vi "TestPowerMeasure.vi"(3 "error in (no error)":errorcluster, 5 "OphirComRef":refnum<k7>) -> (0 "error out":errorcluster, 2 "SerialNumber":string)   [LabVIEW 2012]
uses:
  <vilib>/Analysis/baseanly.llb/Mean (DBL).vi
  <vilib>/Analysis/NI_AALBase.lvlib
panel:
  in  "Measure":bool
  in  "Stop":bool
  out "arrayValue":variant
  out "Array 2":dbl[][](array[numeric])
  out "x != 0?":bool
  out "Array":dbl[](array[numeric])
  out "Errors":dbl[](array[numeric])
  out "mean":dbl format="%.6g"
  out "median":dbl format="%.6g"
  in  "Wavelength":dbl
  in  "Samples":i32
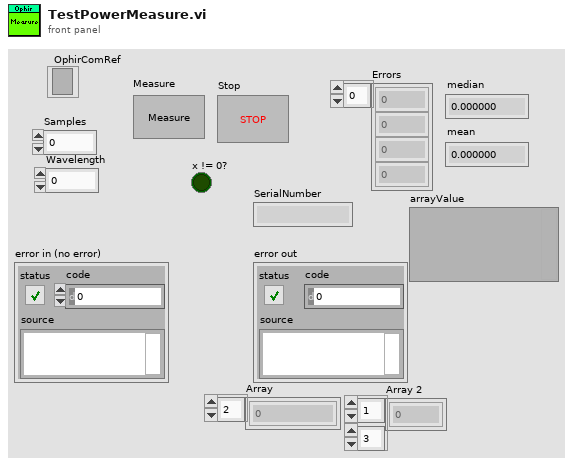
[diagram p1: front panel]
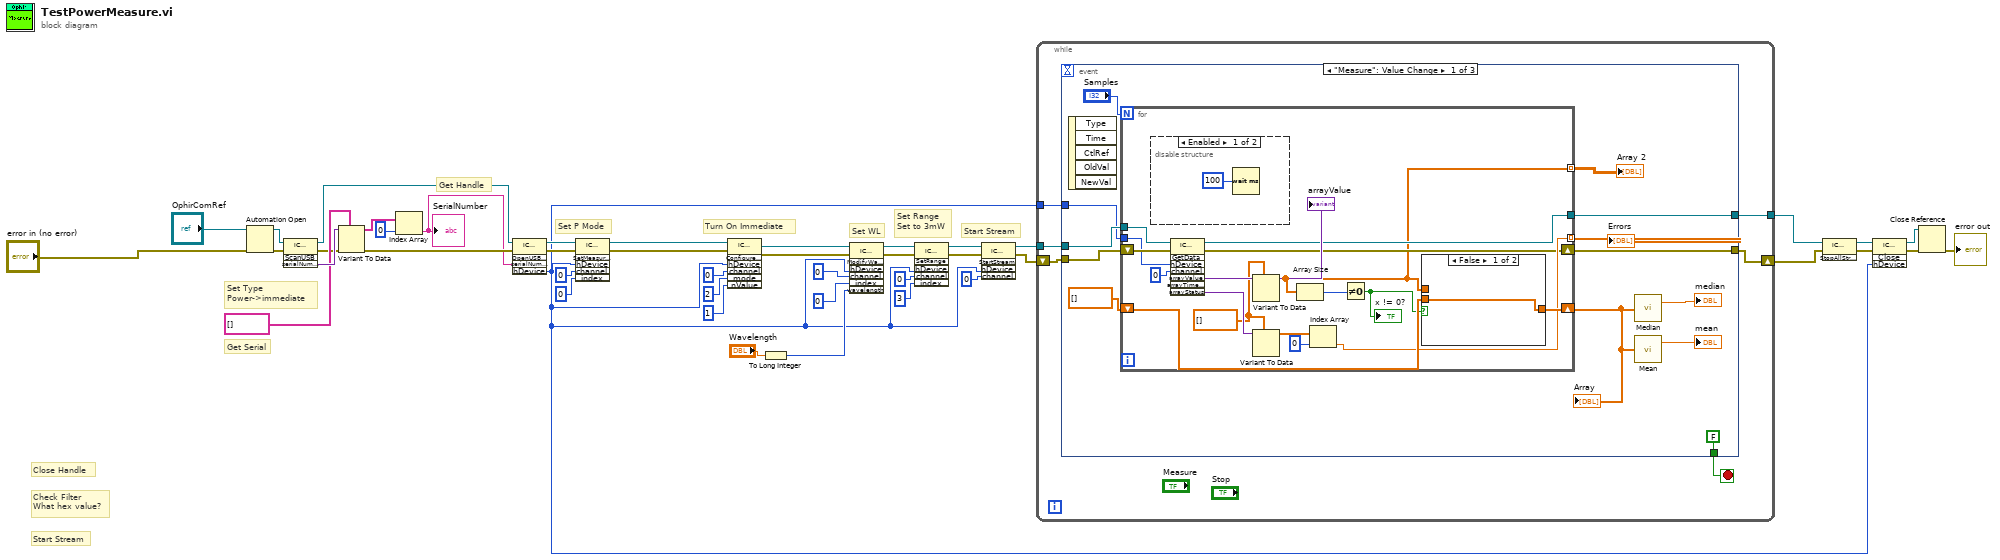
[diagram p0: block diagram]
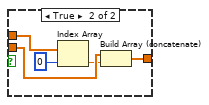
[diagram p3: hidden frame]
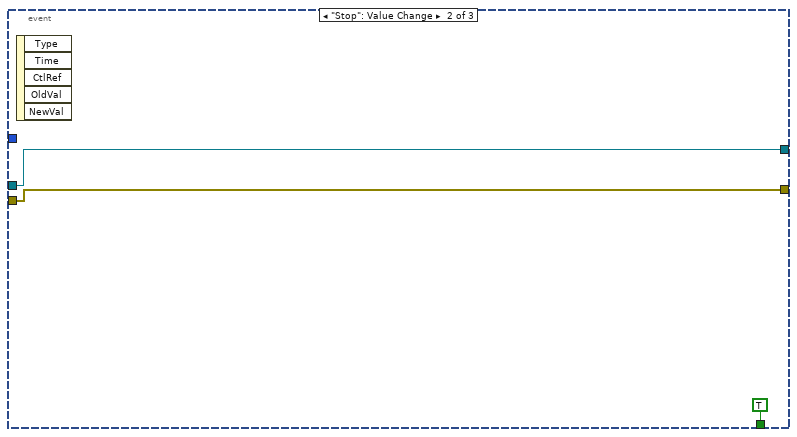
[diagram p4: hidden frame]
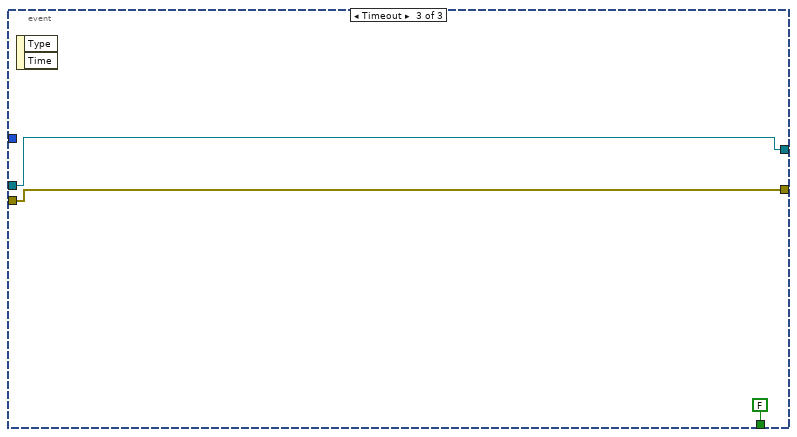
[diagram p5: hidden frame]
diagram:
  # "Start Stream"
  # "Set P Mode"
  # "Turn On Immediate"
  # "Set Type\nPower->immediate"
  # "Close Handle"
  # "Set Range\nSet to 3mW"
  # "Check Filter\nWhat hex value?"
  # "Start Stream"
  # "Get Handle"
  # "Get Serial"
  # "Set WL"
  n1 = Automation Open(error in (no error)="error in (no error)", Automation Refnum="OphirComRef") -> (Automation Refnum=w42:refnum<k7>, error out=w37:errorcluster)  [unwired: 2 in]
  n2 = invoke class="ICoLMMeasurement" method="ScanUSB"(reference=w42, error in=w37) -> (reference out=w34:refnum<k7>, error out=w38:errorcluster, "serialNumbers"=w41:variant)  [unwired: 2 in, 1 out]
  n3 = Variant To Data(error in=w38, type=string[] [], Variant=w41) -> (data=w39:string[], error out=w33:errorcluster)
  n4 = Index Array(array=w39, index=0) -> (element=w32:string)
  "SerialNumber" <- w32
  n5 = invoke class="ICoLMMeasurement" method="OpenUSBDevice"(reference=w34, error in=w33, "serialNumber"=w32) -> (reference out=w18:refnum<k7>, error out=w2:errorcluster, "hDevice"=w1:i32)  [unwired: 2 in, 2 out]
  n6 = invoke class="ICoLMMeasurement" method="SetMeasurementMode"(reference=w18, error in=w2, "hDevice"=w1, "channel"=0, "index"=0) -> (reference out=w4:refnum<k7>, error out=w3:errorcluster)  [unwired: 1 in, 4 out]
  n7 = invoke class="ICoLMMeasurement" method="ConfigureStreamMode"(reference=w4, error in=w3, "hDevice"=w1, "channel"=0 ("mode"), "mode"=2, "nValue"=1) -> (reference out=w7:refnum<k7>, error out=w6:errorcluster)  [unwired: 1 in, 5 out]
  n8 = To Long Integer(number="Wavelength") -> (32bit integer=w26:i32)
  n9 = invoke class="ICoLMMeasurement" method="ModifyWavelength"(reference=w7, error in=w6, "hDevice"=w1, "channel"=0, "index"=0, "wavelength"=w26) -> (reference out=w24:refnum<k7>, error out=w23:errorcluster)  [unwired: 1 in, 5 out]
  n10 = invoke class="ICoLMMeasurement" method="SetRange"(reference=w24, error in=w23, "hDevice"=w1, "channel"=0, "index"=3) -> (reference out=w13:refnum<k7>, error out=w14:errorcluster)  [unwired: 1 in, 4 out]
  n11 = invoke class="ICoLMMeasurement" method="StartStream"(reference=w13, error in=w14, "hDevice"=w1, "channel"=0) -> (reference out=w30:refnum<k7>, error out=w29:errorcluster)  [unwired: 1 in, 3 out]
  n12 = while {
    tunnel: w30 -> [w50]
    tunnel: w1 -> [w47]
    tunnel: [w46] -> w5
    shift-right: [w48] -> w12
    shift-left: w29 -> [w49]
    stop <- w45 stop-if-true
    n13 = event shown="[0] \"Measure\": Value Change" {
      selector: _ -> [_ _ _]
      dyn-events: _ -> [_ _ _]
      timeout: _ -> [_ _ _]
      tunnel: w50 -> [w62 w88 w91]
      tunnel: w49 -> [w61 w89 w92]
      tunnel: [w55 w89 w92] -> w48
      tunnel: w47 -> [w54 _ _]
      tunnel: [w53 w88 w91] -> w46
      tunnel: [FALSE ("Stop") TRUE ("Stop") FALSE ("Stop")] -> w45
      event "Measure": Value Change {
        n14 = event-data() -> ()  [unwired: 1 in, 5 out]
        n15 = for {
          N: "Samples" -> [_]
          tunnel: w62 -> [w80]
          shift-right: [w75] -> w59
          shift-left: dbl[] [] -> [w76]
          tunnel: [w70] -> w56 mode=indexing
          shift-right: [w69] -> w55
          shift-left: w61 -> [w79]
          tunnel: w54 -> [w68]
          tunnel: [w66] -> w53
          tunnel: [w64] -> w52 mode=indexing
          w73 = dbl[] []
          n16 = disable-structure shown="Enabled" {
            frame Enabled {
              n17 = Wait (ms)(milliseconds to wait=u32 100) -> ()  [unwired: 1 out]
            }
            frame Disabled {
            }
          }
          n18 = invoke class="ICoLMMeasurement" method="GetData"(reference=w80, error in=w79, "hDevice"=w68, "channel"=0) -> (reference out=w66:refnum<k7>, error out=w69:errorcluster, "arrayValue"=w78:variant, "arrayStatus"=w74:variant)  [unwired: 4 in, 4 out]
          "arrayValue" <- w78
          n19 = Variant To Data(type=w73, Variant=w78) -> (data=w64:dbl[])  [unwired: 1 in, 1 out]
          n20 = Variant To Data(type=w73, Variant=w74) -> (data=w72:dbl[])  [unwired: 1 in, 1 out]
          n21 = Array Size(array=w64) -> (size(s)=w77:i32)
          n22 = Index Array(array=w72, index=0) -> (element=w70:dbl)
          n23 = Not Equal To 0?(x=w77) -> (x != 0?=w65:bool)
          "x != 0?" <- w65
          n24 = case shown="False" w65 {
            tunnel: w64 -> [_ w87]
            tunnel: w76 -> [w82 w85]
            tunnel: [w82 w83] -> w75
            frame False {
            }
            frame True {
              n25 = Index Array(array=w87, index=0) -> (element=w84:dbl)
              n26 = Build Array (concatenate)(w85, w84) -> (w83:dbl[])
            }
          }
        }
        "Errors" <- w56
        "Array" <- w59
        "Array 2" <- w52
        n27 = call <vilib>:"Median.vi"("X"=w59) -> ("median"=→"median":dbl)  [unwired: 1 out]
        n28 = call-poly <vilib>:"Mean.vi"("X"=w59) -> ("mean"=→"mean":dbl)  [unwired: 1 out]
      }
      event "Stop": Value Change {
        n29 = event-data() -> ()  [unwired: 1 in, 5 out]
      }
      event Timeout {
        n30 = event-data() -> ()  [unwired: 1 in, 2 out]
      }
    }
  }
  n31 = invoke class="ICoLMMeasurement" method="StopAllStreams"(reference=w5, error in=w12) -> (reference out=w11:refnum<k7>, error out=w10:errorcluster)  [unwired: 1 in, 1 out]
  n32 = invoke class="ICoLMMeasurement" method="Close"(reference=w11, error in=w10, "hDevice"=w1) -> (reference out=w8:refnum<k7>, error out=w9:errorcluster)  [unwired: 1 in, 2 out]
  n33 = Close Reference(reference=w8, error in (no error)=w9) -> (error out=→"error out":errorcluster)
